vi "Read StateName.vi"(8 "error in (no error)":errorcluster, 11 "Attribute.Instrument  in":refnum<class "Attribute.Instrument.lvclass">) -> (0 "error out":errorcluster, 2 "StateName":string, 3 "Attribute.Instrument out":refnum<class "Attribute.Instrument.lvclass">)   [LabVIEW 2019, in "Instrument Attributes.lvlib" / "Attribute.Instrument.lvclass"]
uses:
  Attribute.Instrument.lvclass
  Attribute.Instrument.lvclass/Attribute.Instrument.ctl
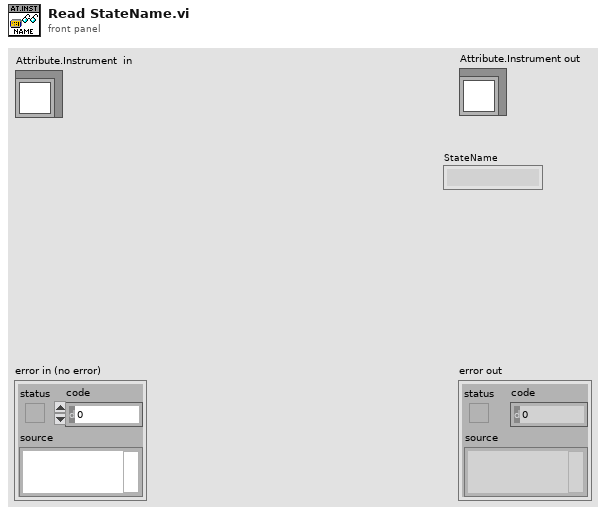
[diagram p1: front panel]
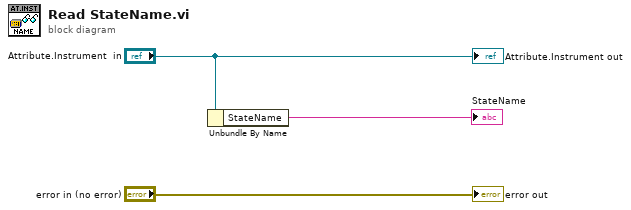
[diagram p0: block diagram]
diagram:
  n1 = Unbundle By Name("Attribute.Instrument  in") -> ("StateName"=→"StateName":string)
  "error out" <- "error in (no error)"
  "Attribute.Instrument out" <- "Attribute.Instrument  in"
